vi "TrapsMachMitteln-11-15.vi"(0 "FPGA VI Reference In":refnum<k20>, 1 "Traps/MachKoeff2":dbl[](array[numeric]), 2 "Traps/MachKoeff1":dbl[](array[numeric]), 3 "Traps/MachKoeff0":dbl[](array[numeric]), 4 "error in":errorcluster) -> (5 "error out":errorcluster)   [LabVIEW 2010]
uses:
  <vilib>/rvi/interface/nirviReadWriteControl/nirviReadWriteControl.xnode
  C:/Users/HAGAR-IV/Desktop/Zeugs/markus/version feb 2012/FPGA Bitfiles/pertrasgcfpga2_FPGATarget_FPGA-Programm-11_875D3646.lvbitx
  C:/Users/HAGAR-IV/Desktop/Zeugs/Johnny/pertrasgc fpga/FPGA-Programm-11-15.vi
  <vilib>/rvi/interface/common/niFpgaNodeNameForErrorReporting.ctl
  <vilib>/rvi/errors/niLvFpgaWhatHappensToTopLevelVI.ctl
  GVTrapsMachs.vi
  <vilib>/Utility/error.llb/Error Cluster From Error Code.vi
  <vilib>/rvi/errors/niLvFpgaAdjustHostInterfaceError.vi
  NiFpgaLv.dll
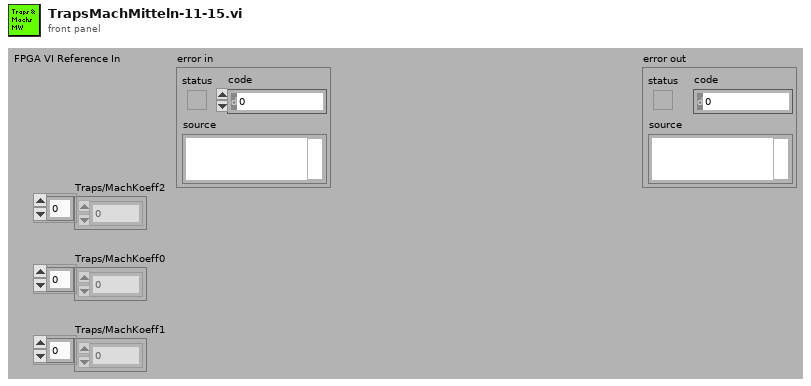
[diagram p1: front panel]
types:
  T1 = typedef "niFpgaNodeNameForErrorReporting.ctl" = enum16{"Open FPGA VI Reference", "Read/Write Control", "Invoke Method: Abort", "Invoke Method: Acknowledge IRQ", "Invoke Method: Download", "Invoke Method: FIFO.Configure", "Invoke Method: FIFO.Read", "Invoke Method: FIFO.Start", "Invoke Method: FIFO.Stop", "Invoke Method: FIFO.Write", "Invoke Method: Reset", "Invoke Method: Run", "Invoke Method: Wait on IRQ", "Close FPGA VI Reference"}
  T2 = typedef "niLvFpgaWhatHappensToTopLevelVI.ctl" = enum16{"top level VI scripted behind XNode", "top level VI inlined behind XNode"}
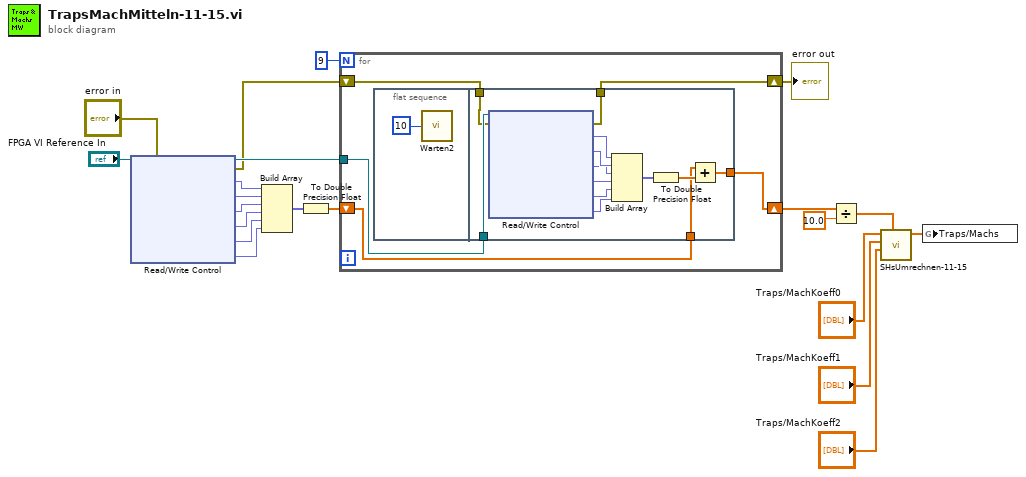
[diagram p0: block diagram]
diagram:
  n1 = xnode "Read/Write Control"("FPGA VI Reference In"="FPGA VI Reference In", "error in"="error in") -> ("FPGA VI Reference Out"=w20:refnum<k20>, "error out"=w2:errorcluster, "UTemp[V]Trap1"=w14:fxp<+/-,16,4>, "UTemp[V]Trap2"=w13:fxp<+/-,16,4>, "U[V]PreMach1"=w12:fxp<+/-,16,4>, "U[V]PreMach2"=w11:fxp<+/-,16,4>, "U[V]MainMach1"=w10:fxp<+/-,16,4>, "U[V]MainMach2"=w9:fxp<+/-,16,4>)
  n2 = Build Array(w14, w13, w12, w11, w10, w9) -> (w16:fxp<+/-,16,4>[])
  n3 = To Double Precision Float(number=w16) -> (double precision float=w21:dbl[])
  n4 = for {
    N: 9 -> [_]
    tunnel: w20 -> [w26]
    shift-right: [w24] -> w18
    shift-left: w21 -> [w25]
    shift-right: [w22] -> w1
    shift-left: w2 -> [w23]
    n5 = flat-sequence {
      tunnel: w26 -> [w36]
      tunnel: w25 -> [w38]
      tunnel: [w37] -> w24
      tunnel: w23 -> [w29]
      tunnel: [w28] -> w22
      frame #0 {
        n6 = call "Warten2"("Count(mSec)"=u32 10) -> ()  [unwired: 1 out]
      }
      frame #1 {
        n7 = xnode "Read/Write Control"("FPGA VI Reference In"=w36, "error in"=w29) -> ("error out"=w28:errorcluster, "UTemp[V]Trap1"=w35:fxp<+/-,16,4>, "UTemp[V]Trap2"=w34:fxp<+/-,16,4>, "U[V]PreMach1"=w33:fxp<+/-,16,4>, "U[V]PreMach2"=w32:fxp<+/-,16,4>, "U[V]MainMach1"=w31:fxp<+/-,16,4>, "U[V]MainMach2"=w30:fxp<+/-,16,4>)  [unwired: 1 out]
        n8 = Build Array(w35, w34, w33, w32, w31, w30) -> (w40:fxp<+/-,16,4>[])
        n9 = To Double Precision Float(number=w40) -> (double precision float=w39:dbl[])
        n10 = Add(x=w38, y=w39) -> (x+y=w37:dbl[])
      }
    }
  }
  "error out" <- w1
  n11 = Divide(x=w18, y=10.0) -> (x/y=w5:dbl[])
  n12 = call "SHsUmrechnen-11-15.vi"("SpannungenSH[V]"=w5, "Traps/MachKoeff2"="Traps/MachKoeff2", "Traps/MachKoeff1"="Traps/MachKoeff1", "Traps/MachKoeff0"="Traps/MachKoeff0") -> ("TemperaturenSH[°C]"=w4:dbl[])  [unwired: 6 in, 1 out]
  n13 = global write "GVTrapsMachs.vi" "Traps/Machs"(w4) -> ()
